vi "niDTS WLAN Tx Test INC Default Limits.vi"() -> ()   [LabVIEW 2015, in "niDTS WLAN.lvlib"]
uses:
  niDTS WLAN.lvlib
  Results/niDTS Tx RES INC EVM.ctl
  niDTS WLAN Tx Test INC OBW Results.ctl
  niDTS WLAN Tx Test INC TXP Result SINGLE.ctl
  Results/niDTS Tx RES INC SEM FSEGemts.ctl
  Results/niDTS Tx RES INC SEM Margin.ctl
panel:
  out "Default USL OFDM Impairments":T1={"SampleClockOffset"=inf, "CarrierFrequencyOffset"=inf, "AvgRmsComPilotErr"=inf, "RmsPhaseNoise"=inf, "ChannelData"=[{"CarrierFrequencyOffset"=999999999, "AvgRmsComPilotErr"=inf, "RmsPhaseNoise"=inf, "ChannelData"=inf, "ChannelIndex"=inf}]}
  out "Default LSL OFDM Impairments":T1={"SampleClockOffset"=-inf, "CarrierFrequencyOffset"=-inf, "AvgRmsComPilotErr"=-inf, "RmsPhaseNoise"=-inf, "ChannelData"=[{"CarrierFrequencyOffset"=-999999999, "AvgRmsComPilotErr"=-inf, "RmsPhaseNoise"=-inf, "ChannelData"=-inf, "ChannelIndex"=-inf}]}
  out "Defaukt USL SEM Margin 802.11ac":T2={"Chain Index"=100, "Worst Case Out Of Band Margin (dB)"=inf, "Worst Case Out Of Band Frequency (Hz)"=inf, "Violation (%)"=inf}
  in  "Default USL SEM FSEG 802.11ac":T3={"Chain Index"=100, "Number Of Segments"=100, "Frequecy Segment Results"={"Segment Index"=100, "Margin (dB)"=inf, "Reference Level (dBm/Hz)"=inf, "Worst Case Frequency (Hz)"=inf}}
  out "Defaukt LSL SEM Margin 802.11ac":T2={"Chain Index"=0, "Worst Case Out Of Band Margin (dB)"=-inf, "Worst Case Out Of Band Frequency (Hz)"=-inf, "Violation (%)"=-inf}
  in  "Default LSL SEM FSEG 802.11ac":T3={"Chain Index"=0, "Number Of Segments"=0, "Frequecy Segment Results"={"Segment Index"=0, "Margin (dB)"=-inf, "Reference Level (dBm/Hz)"=-inf, "Worst Case Frequency (Hz)"=-inf}}
  out "Defaukt USL SEM Margin 802.11n":T2={"Chain Index"=100, "Worst Case Out Of Band Margin (dB)"=inf, "Worst Case Out Of Band Frequency (Hz)"=inf, "Violation (%)"=inf}
  in  "Default USL SEM FSEG 802.11n":T3={"Chain Index"=100, "Number Of Segments"=100, "Frequecy Segment Results"={"Segment Index"=100, "Margin (dB)"=inf, "Reference Level (dBm/Hz)"=inf, "Worst Case Frequency (Hz)"=inf}}
  out "Defaukt LSL SEM Margin 802.11n":T2={"Chain Index"=0, "Worst Case Out Of Band Margin (dB)"=-inf, "Worst Case Out Of Band Frequency (Hz)"=-inf, "Violation (%)"=-inf}
  in  "Default LSL SEM FSEG 802.11n":T3={"Chain Index"=0, "Number Of Segments"=0, "Frequecy Segment Results"={"Segment Index"=0, "Margin (dB)"=-inf, "Reference Level (dBm/Hz)"=-inf, "Worst Case Frequency (Hz)"=-inf}}
  out "Defaukt USL SEM Margin 802.11a/g":T2={"Chain Index"=100, "Worst Case Out Of Band Margin (dB)"=inf, "Worst Case Out Of Band Frequency (Hz)"=inf, "Violation (%)"=inf}
  in  "Default USL SEM FSEG 802.11a/g":T3={"Chain Index"=100, "Number Of Segments"=100, "Frequecy Segment Results"={"Segment Index"=100, "Margin (dB)"=inf, "Reference Level (dBm/Hz)"=inf, "Worst Case Frequency (Hz)"=inf}}
  out "Defaukt LSL SEM Margin 802.11a/g":T2={"Chain Index"=0, "Worst Case Out Of Band Margin (dB)"=-inf, "Worst Case Out Of Band Frequency (Hz)"=-inf, "Violation (%)"=-inf}
  in  "Default LSL SEM FSEG 802.11a/g":T3={"Chain Index"=0, "Number Of Segments"=0, "Frequecy Segment Results"={"Segment Index"=0, "Margin (dB)"=-inf, "Reference Level (dBm/Hz)"=-inf, "Worst Case Frequency (Hz)"=-inf}}
  in  "Default Relative USL TXP 802.11ac":T4={"Chain Index"=100.0, "Average Power (dBm)"=inf, "Peak Power (dBm)"=inf, "Avg Power w Gap (dBm)"=inf}
  in  "Default Relative LSL TXP 802.11ac":T4={"Chain Index"=0.0, "Average Power (dBm)"=-inf, "Peak Power (dBm)"=-inf, "Avg Power w Gap (dBm)"=-inf}
  in  "Default Relative USL OBW 802.11ac":T5={"Chain Index"=100.0, "OBW (Hz)"=inf, "Start Frequency (Hz)"=inf, "Stop Frequency (Hz)"=inf} {"Stop Frequency (Hz)" format="%#_4p"; "Start Frequency (Hz)" format="%#_4p"; "OBW (Hz)" format="%#_4p"}
  in  "Default Relative LSL OBW 802.11ac":T5={"Chain Index"=0.0, "OBW (Hz)"=-inf, "Start Frequency (Hz)"=-inf, "Stop Frequency (Hz)"=-inf} {"Stop Frequency (Hz)" format="%#_4p"; "Start Frequency (Hz)" format="%#_4p"; "OBW (Hz)" format="%#_4p"}
  in  "Default USL EVM 802.11ac":T6={"Stream Index"=100, "Packet (dB)"=0.0, "Pilot (dB)"=0.0, "Data (dB)"=0.0}
  in  "Default LSL EVM 802.11ac":T6={"Stream Index"=0, "Packet (dB)"=-100.0, "Pilot (dB)"=-100.0, "Data (dB)"=-100.0}
  in  "Default Relative USL TXP 802.11n":T4={"Chain Index"=100.0, "Average Power (dBm)"=inf, "Peak Power (dBm)"=inf, "Avg Power w Gap (dBm)"=inf}
  in  "Default Relative LSL TXP 802.11n":T4={"Chain Index"=0.0, "Average Power (dBm)"=-inf, "Peak Power (dBm)"=-inf, "Avg Power w Gap (dBm)"=-inf}
  in  "Default Relative USL OBW 802.11n":T5={"Chain Index"=100.0, "OBW (Hz)"=inf, "Start Frequency (Hz)"=inf, "Stop Frequency (Hz)"=inf} {"Stop Frequency (Hz)" format="%#_4p"; "Start Frequency (Hz)" format="%#_4p"; "OBW (Hz)" format="%#_4p"}
  in  "Default Relative LSL OBW 802.11n":T5={"Chain Index"=0.0, "OBW (Hz)"=-inf, "Start Frequency (Hz)"=-inf, "Stop Frequency (Hz)"=-inf} {"Stop Frequency (Hz)" format="%#_4p"; "Start Frequency (Hz)" format="%#_4p"; "OBW (Hz)" format="%#_4p"}
  in  "Default USL EVM 802.11n":T6={"Stream Index"=100, "Packet (dB)"=0.0, "Pilot (dB)"=0.0, "Data (dB)"=0.0}
  in  "Default LSL EVM 802.11n":T6={"Stream Index"=0, "Packet (dB)"=-100.0, "Pilot (dB)"=-100.0, "Data (dB)"=-100.0}
  in  "Default Relative USL TXP 802.11a/g":T4={"Chain Index"=100.0, "Average Power (dBm)"=inf, "Peak Power (dBm)"=inf, "Avg Power w Gap (dBm)"=inf}
  in  "Default Relative LSL TXP 802.11a/g":T4={"Chain Index"=0.0, "Average Power (dBm)"=-inf, "Peak Power (dBm)"=-inf, "Avg Power w Gap (dBm)"=-inf}
  in  "Default Relative USL OBW 802.11a/g":T5={"Chain Index"=100.0, "OBW (Hz)"=inf, "Start Frequency (Hz)"=inf, "Stop Frequency (Hz)"=inf} {"Stop Frequency (Hz)" format="%#_4p"; "Start Frequency (Hz)" format="%#_4p"; "OBW (Hz)" format="%#_4p"}
  in  "Default Relative LSL OBW 802.11a/g":T5={"Chain Index"=0.0, "OBW (Hz)"=-inf, "Start Frequency (Hz)"=-inf, "Stop Frequency (Hz)"=-inf} {"Stop Frequency (Hz)" format="%#_4p"; "Start Frequency (Hz)" format="%#_4p"; "OBW (Hz)" format="%#_4p"}
  in  "Default USL EVM 802.11a/g":T6={"Stream Index"=100, "Packet (dB)"=0.0, "Pilot (dB)"=0.0, "Data (dB)"=0.0}
  in  "Default LSL EVM 802.11a/g":T6={"Stream Index"=0, "Packet (dB)"=-100.0, "Pilot (dB)"=-100.0, "Data (dB)"=-100.0}
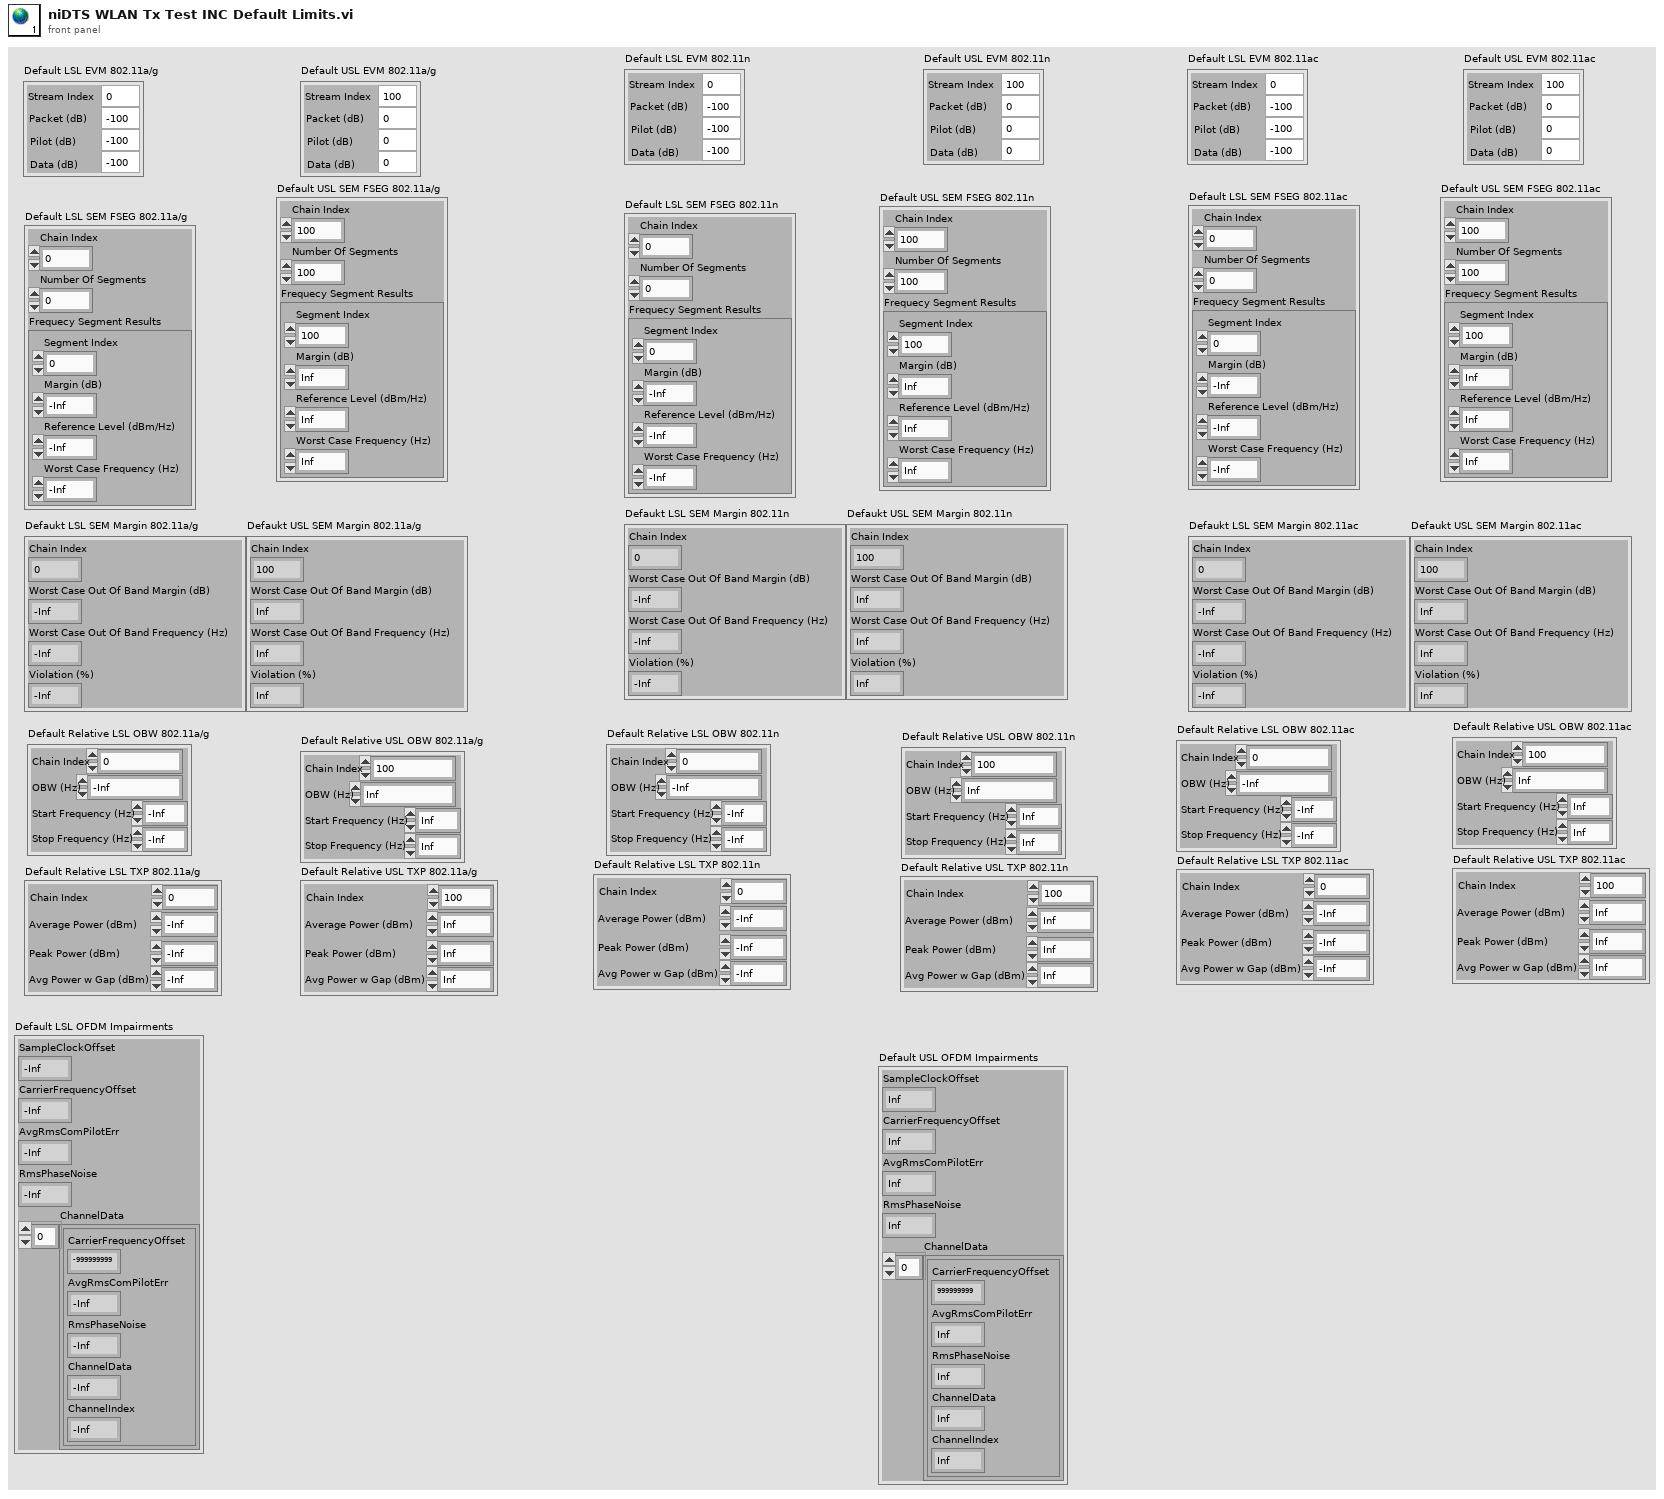
[diagram p1: front panel]
types:
  T1 = cluster{"SampleClockOffset":dbl, "CarrierFrequencyOffset":dbl, "AvgRmsComPilotErr":dbl, "RmsPhaseNoise":dbl, "ChannelData":cluster{"CarrierFrequencyOffset":i32, "AvgRmsComPilotErr":dbl, "RmsPhaseNoise":dbl, "ChannelData":dbl, "ChannelIndex":dbl}[]}
  T2 = typedef "niDTS WLAN.lvlib/niDTS Tx RES INC SEM Margin.ctl" = cluster{"Chain Index":i32, "Worst Case Out Of Band Margin (dB)":dbl, "Worst Case Out Of Band Frequency (Hz)":dbl, "Violation (%)":dbl}
  T3 = typedef "niDTS WLAN.lvlib/niDTS Tx RES INC SEM FSEGemts.ctl" = cluster{"Chain Index":i32, "Number Of Segments":i32, "Frequecy Segment Results":cluster{"Segment Index":i32, "Margin (dB)":dbl, "Reference Level (dBm/Hz)":dbl, "Worst Case Frequency (Hz)":dbl}}
  T4 = typedef "niDTS WLAN.lvlib/niDTS WLAN Tx Test INC TXP Result SINGLE.ctl" = cluster{"Chain Index":dbl, "Average Power (dBm)":dbl, "Peak Power (dBm)":dbl, "Avg Power w Gap (dBm)":dbl}
  T5 = typedef "niDTS WLAN.lvlib/niDTS WLAN Tx Test INC OBW Results.ctl" = cluster{"Chain Index":dbl, "OBW (Hz)":dbl, "Start Frequency (Hz)":dbl, "Stop Frequency (Hz)":dbl}
  T6 = typedef "niDTS WLAN.lvlib/niDTS Tx RES INC EVM.ctl" = cluster{"Stream Index":i32, "Packet (dB)":dbl, "Pilot (dB)":dbl, "Data (dB)":dbl}
diagram:
